vi "Danger Array_Calculate Attack Points.vi"(0 "Move Map":i32[][](array[numeric]), 4 "Round":i32, 6 "Team Index":i32, 7 "Danger Map":i32[][](array[numeric]), 8 "Calulate Multiple":i32=50, 9 "Board Size":i32, 10 "Danger Column":i32[](array[numeric]), 11 "Danger Row":i32[](array[numeric])) -> (2 "Danger Column Out":i32[](array[numeric]), 3 "Danger Row Out":i32[](array[numeric]), 5 "Danger Threshold":i32)   [LabVIEW 2017, in "AntFarm_MB.lvclass"]
uses:
  AntFarm_MB.lvclass
  SubVIs/Read-Only Stats.vi
  Square/Square.lvclass
panel:
  in  "Danger Threshold Array":i32[](array[numeric])=[110, 100, 90, 80]
  in  "Point Count Set Array":i32[](array[numeric])=[64, 32, 16, 8]
  in  "Percent Lookup Array":dbl[](array[numeric])=[0.8, 0.6, 0.4, 0.3]
  out "Point Count":i32
  out "score":i32[](array[numeric])
  out "Percent":dbl
  out "Squares":i32
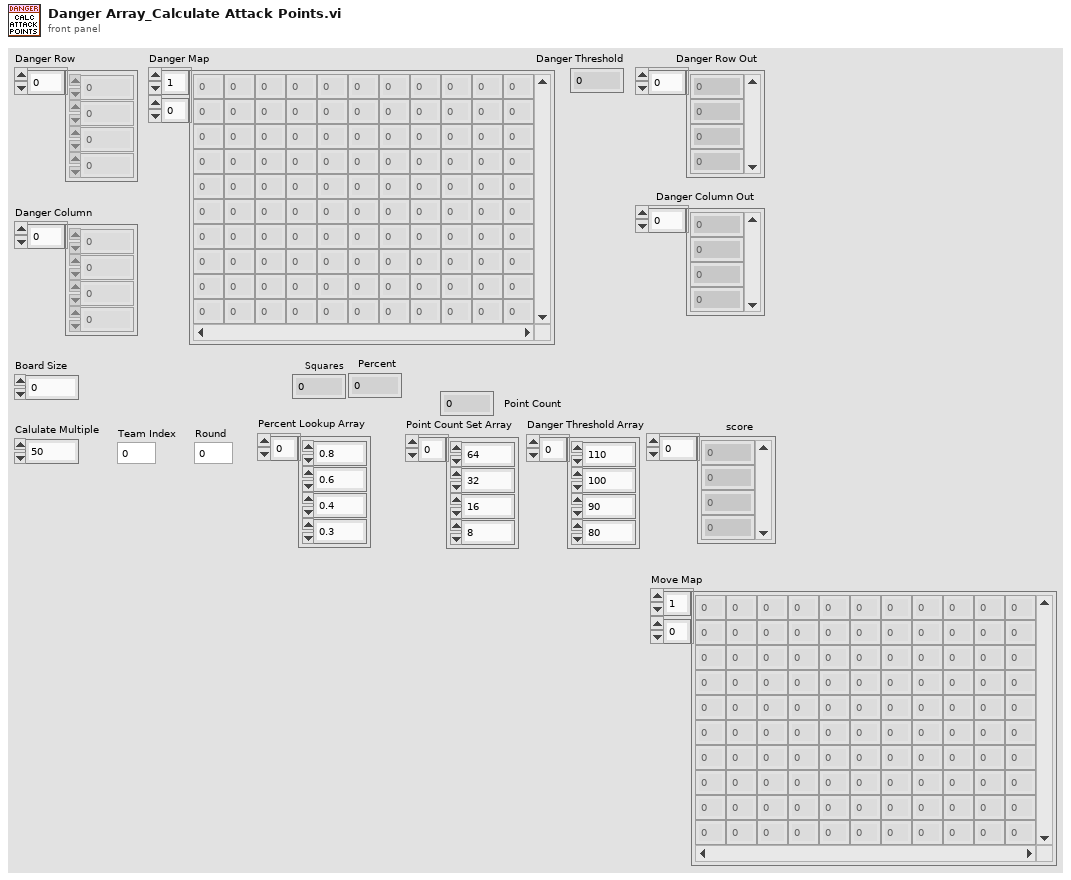
[diagram p1: front panel]
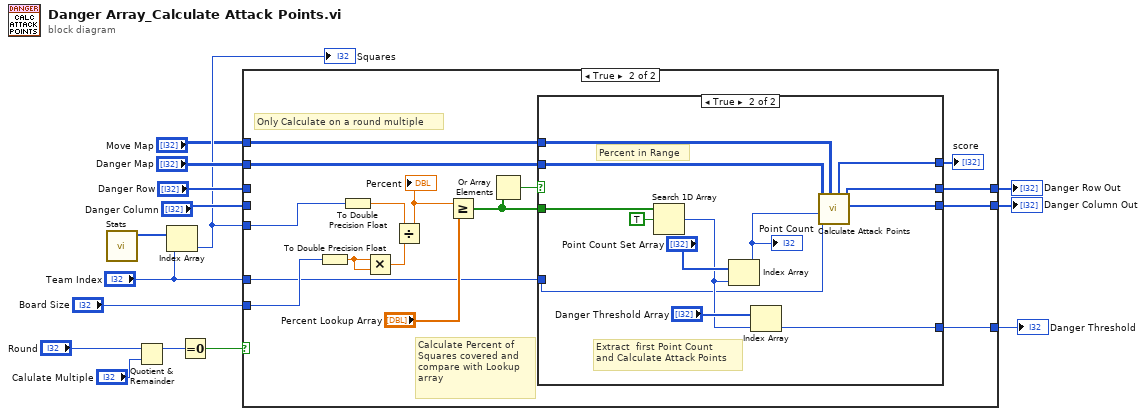
[diagram p0: block diagram]
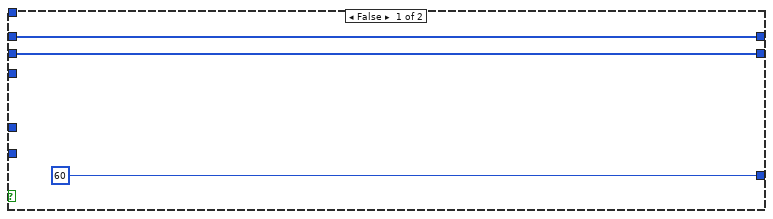
[diagram p2: hidden frame]
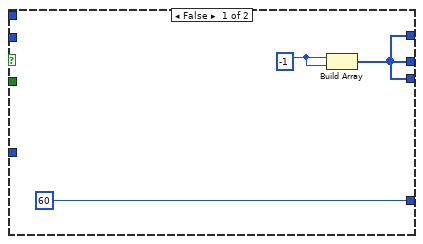
[diagram p3: hidden frame]
diagram:
  n1 = call "Stats.vi"() -> ("Squares"=w6:i32[])  [unwired: 7 in, 4 out]
  n2 = Quotient & Remainder(x="Round", y="Calulate Multiple") -> (x-y*floor(x/y)=w11:i32)  [unwired: 1 out]
  n3 = Index Array(array=w6, index="Team Index") -> (element=w5:i32)
  "Squares" <- w5
  n4 = Equal To 0?(x=w11) -> (x = 0?=w10:bool)
  n5 = case shown="True" w10 {
    tunnel: [w17 w33] -> w15
    tunnel: [w18 w32] -> w14
    tunnel: "Danger Row" -> [w18 _]
    tunnel: "Danger Column" -> [w17 _]
    tunnel: "Danger Map" -> [_ w30]
    tunnel: w5 -> [_ w29]
    tunnel: "Board Size" -> [_ w28]
    tunnel: [60 ("x*y") w21] -> w3
    tunnel: "Move Map" -> [_ w20]
    tunnel: "Team Index" -> [_ w19]
    frame False {
    }
    frame True {
      # "Calculate Percent of\nSquares covered and\ncompare with Lookup\narray"
      # "Only Calculate on a round multiple"
      n6 = To Double Precision Float(number=w28) -> (double precision float=w34:dbl)
      n7 = To Double Precision Float(number=w29) -> (double precision float=w27:dbl)
      n8 = Multiply(x=w34, y=w34) -> (x*y=w26:dbl)
      n9 = Divide(x=w27, y=w26) -> (x/y=w22:dbl)
      "Percent" <- w22
      n10 = Greater Or Equal?(x=w22, y="Percent Lookup Array") -> (x >= y?=w23:bool[])
      n11 = Or Array Elements(Boolean array=w23) -> (logical OR=w24:bool)
      n12 = case shown="True" w24 {
        tunnel: [w36 w50] -> w32
        tunnel: [w36 w49] -> w33
        tunnel: w30 -> [_ w48]
        tunnel: [w36 w47] -> w31
        tunnel: w23 -> [_ w46]
        tunnel: [60 ("x*y") w40] -> w21
        tunnel: w20 -> [_ w39]
        tunnel: w19 -> [_ w38]
        frame False {
          w37 = -1 ("Danger Row")
          n13 = Build Array(w37, w37) -> (w36:i32[])
        }
        frame True {
          # "Extract  first Point Count\nand Calculate Attack Points"
          # "Percent in Range"
          n14 = Search 1D Array(1D array=w46, element=TRUE) -> (index of element=w41:i32)  [unwired: 1 in]
          n15 = Index Array(array="Point Count Set Array", index=w41) -> (element=w43:i32)
          "Point Count" <- w43
          n16 = Index Array(array="Danger Threshold Array", index=w41) -> (element=w40:i32)
          n17 = call "Calculate Attack Points.vi"("Move Map"=w39, "Team Index"=w38, "Max Atack Points"=w43, "Danger Map"=w48) -> ("Danger Columns Out"=w49:i32[], "Danger Rows Out"=w50:i32[], "Scores Out"=w47:i32[])  [unwired: 5 in]
        }
      }
      "score" <- w31
    }
  }
  "Danger Column Out" <- w15
  "Danger Row Out" <- w14
  "Danger Threshold" <- w3
